vi "AM Do Channels Parsing.vi"(11 "Current Status":u8[](array[numeric])) -> (1 "DO 3W":bool[](array[boolean]), 3 "DO ON-OFF":bool[](array[boolean]))   [LabVIEW 2020, in "Motion.lvlib"]
uses:
  Motion.lvlib
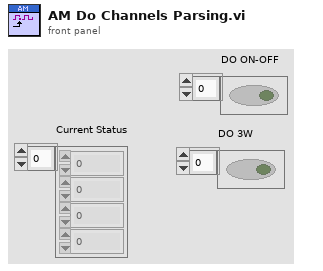
[diagram p1: front panel]
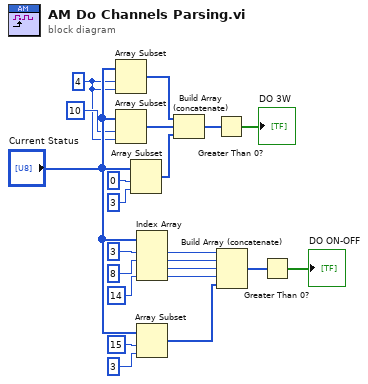
[diagram p0: block diagram]
diagram:
  w1 = 4 ("index")
  n1 = Array Subset(array="Current Status", index=w1, length=w1) -> (w5:u8[])
  n2 = Array Subset(array="Current Status", index=10, length=w1) -> (w6:u8[])
  n3 = Array Subset(array="Current Status", index=0, length=3) -> (w7:u8[])
  n4 = Index Array(array="Current Status", index #1=3 ("index"), index #2=8 ("index"), index #4=14 ("index")) -> (element #1=w17:u8, element #2=w18:u8, element #3=w19:u8, element #4=w20:u8)  [unwired: 1 in]
  n5 = Array Subset(array="Current Status", index=15, length=3) -> (w21:u8[])
  n6 = Build Array (concatenate)(w5, w6, w7) -> (w8:u8[])
  n7 = Greater Than 0?(x=w8) -> (x > 0?=→"DO 3W":bool[])
  n8 = Build Array (concatenate)(w17, w18, w19, w20, w21) -> (w16:u8[])
  n9 = Greater Than 0?(x=w16) -> (x > 0?=→"DO ON-OFF":bool[])
